vi "ReCalc_V0.15.vi"(3 "Berechnen":bool, 4 "Datenspeicher":T2) -> ()   [LabVIEW 2014]
uses:
  <vilib>/Utility/miscctls.llb/LVPointTypeDef.ctl
  <vilib>/Utility/xml.llb/Read From XML File(string).vi
  <vilib>/Analysis/3filter.llb/IIR Filter (DBL).vi
  <vilib>/Analysis/NI_AALBase.lvlib
  <vilib>/Analysis/NI_AALPro.lvlib
panel:
  out "Fahrzeugdaten":string
  out "Überlagerung":bool
  in  "Überlagern":bool
  out "Übersetzung ermitteln aus":T1(ring)
  in  "Speichern":bool
  out "Reifenumfang [m]":dbl=1.222
  out "Getriebe [1:]":dbl=5.343
  out "Zündung [Imp/U]":u8=1
  out "Rollengeber [Inkr/U]":u16=200
  out "Luftdruck [mbar]":dbl=1013.0
  out "Luftfeuchtigkeit [%]":dbl=50.0
  out "Lufttemperatur [°C]":dbl=20.0
  in  "Stopp":bool
  in  "Rollenträgheit [kgm²]":dbl=0.402
  in  "Polynom":u8=15
  in  "Gl. Mittelwert":u8=35
  in  "Differenzenquotient":u8=12
  in  "n vom Gas [1/min]":dbl=5000.0
  out "Rollenumfang [m]":dbl=0.613 format="%.3f"
  out "Datum, Zeit":string
  out "Untersetzung aus:":dbl=2.68 format="%.2f"
  in  "Drucken":bool
  out "Pmax":string
  out "Ergebnis":string
  out "XY-Graph":cluster{dbl[], dbl[]}[](graph)
  in  "Öffnen":bool
  out "korr":dbl
  out "[s]":dbl=5.0
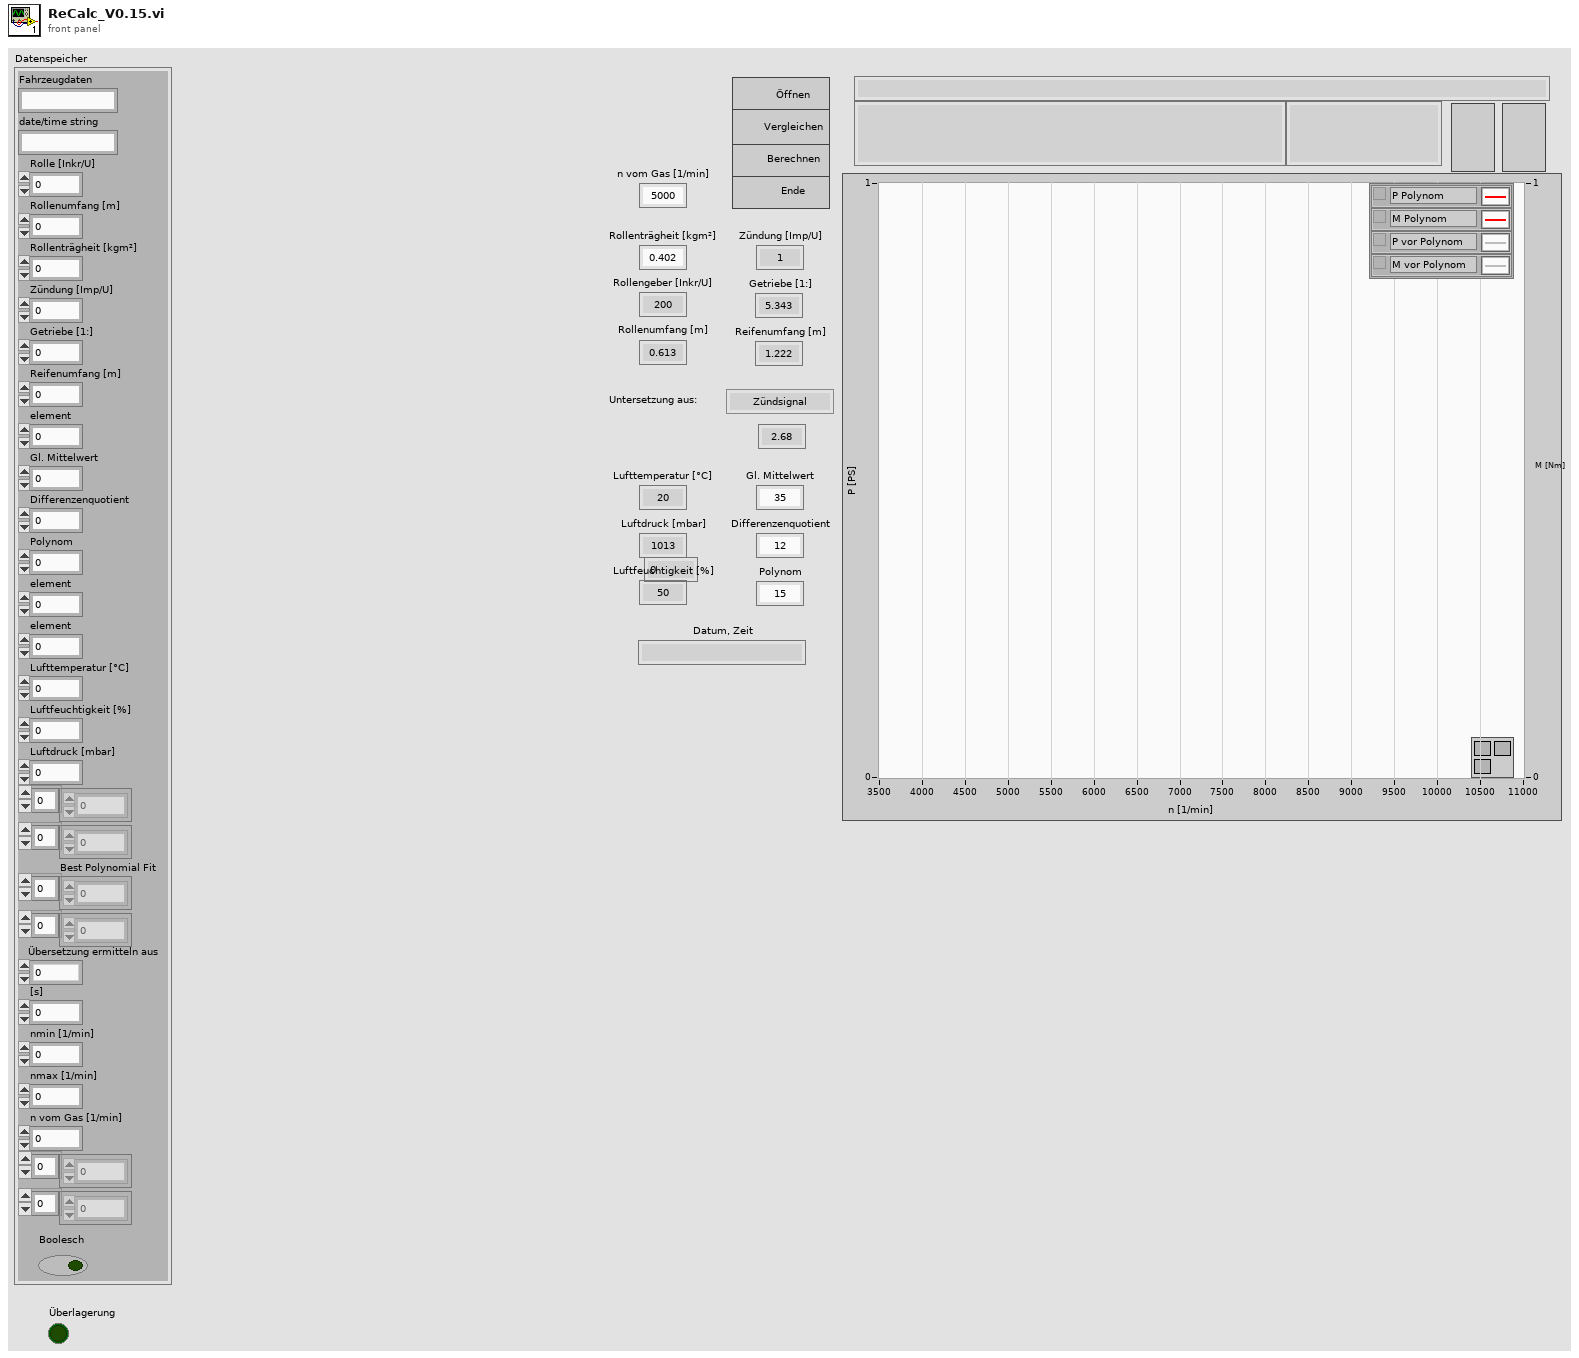
[diagram p1: front panel]
types:
  T1 = enum8{"Zündsignal", "Getriebe & Reifen", "nKuWe / nRolle :"}
  T2 = cluster{"Fahrzeugdaten":string, "date/time string":string, "Rolle [Inkr/U]":u16, "Rollenumfang [m]":dbl, "Rollenträgheit [kgm²]":dbl, "Zündung [Imp/U]":u8, "Getriebe [1:]":dbl, "Reifenumfang [m] ":dbl, "element":dbl, "Gl. Mittelwert":u8, "Differenzenquotient":u8, "Polynom":u8, "element":dbl, "element":dbl, "Lufttemperatur [°C]":dbl, "Luftfeuchtigkeit [%]":dbl, "Luftdruck [mbar]":dbl, dbl[], dbl[], "Best Polynomial Fit":dbl[], dbl[], "Übersetzung ermitteln aus":u8, "[s]":dbl, "nmin [1/min]":dbl, "nmax [1/min]":dbl, "n vom Gas [1/min]":dbl, dbl[], i32[], "Boolesch":bool}
  T3 = typedef "LVPointTypeDef.ctl" = cluster{"Horizontal":i16, "Vertical":i16}
  T4 = enum16{"Kleinste Quadrate", "Kleinestes absolutes Reiduum", "Biquadrat"}
  T5 = enum8{"Enabled", "Disabled", "Disabled and Grayed Out"}
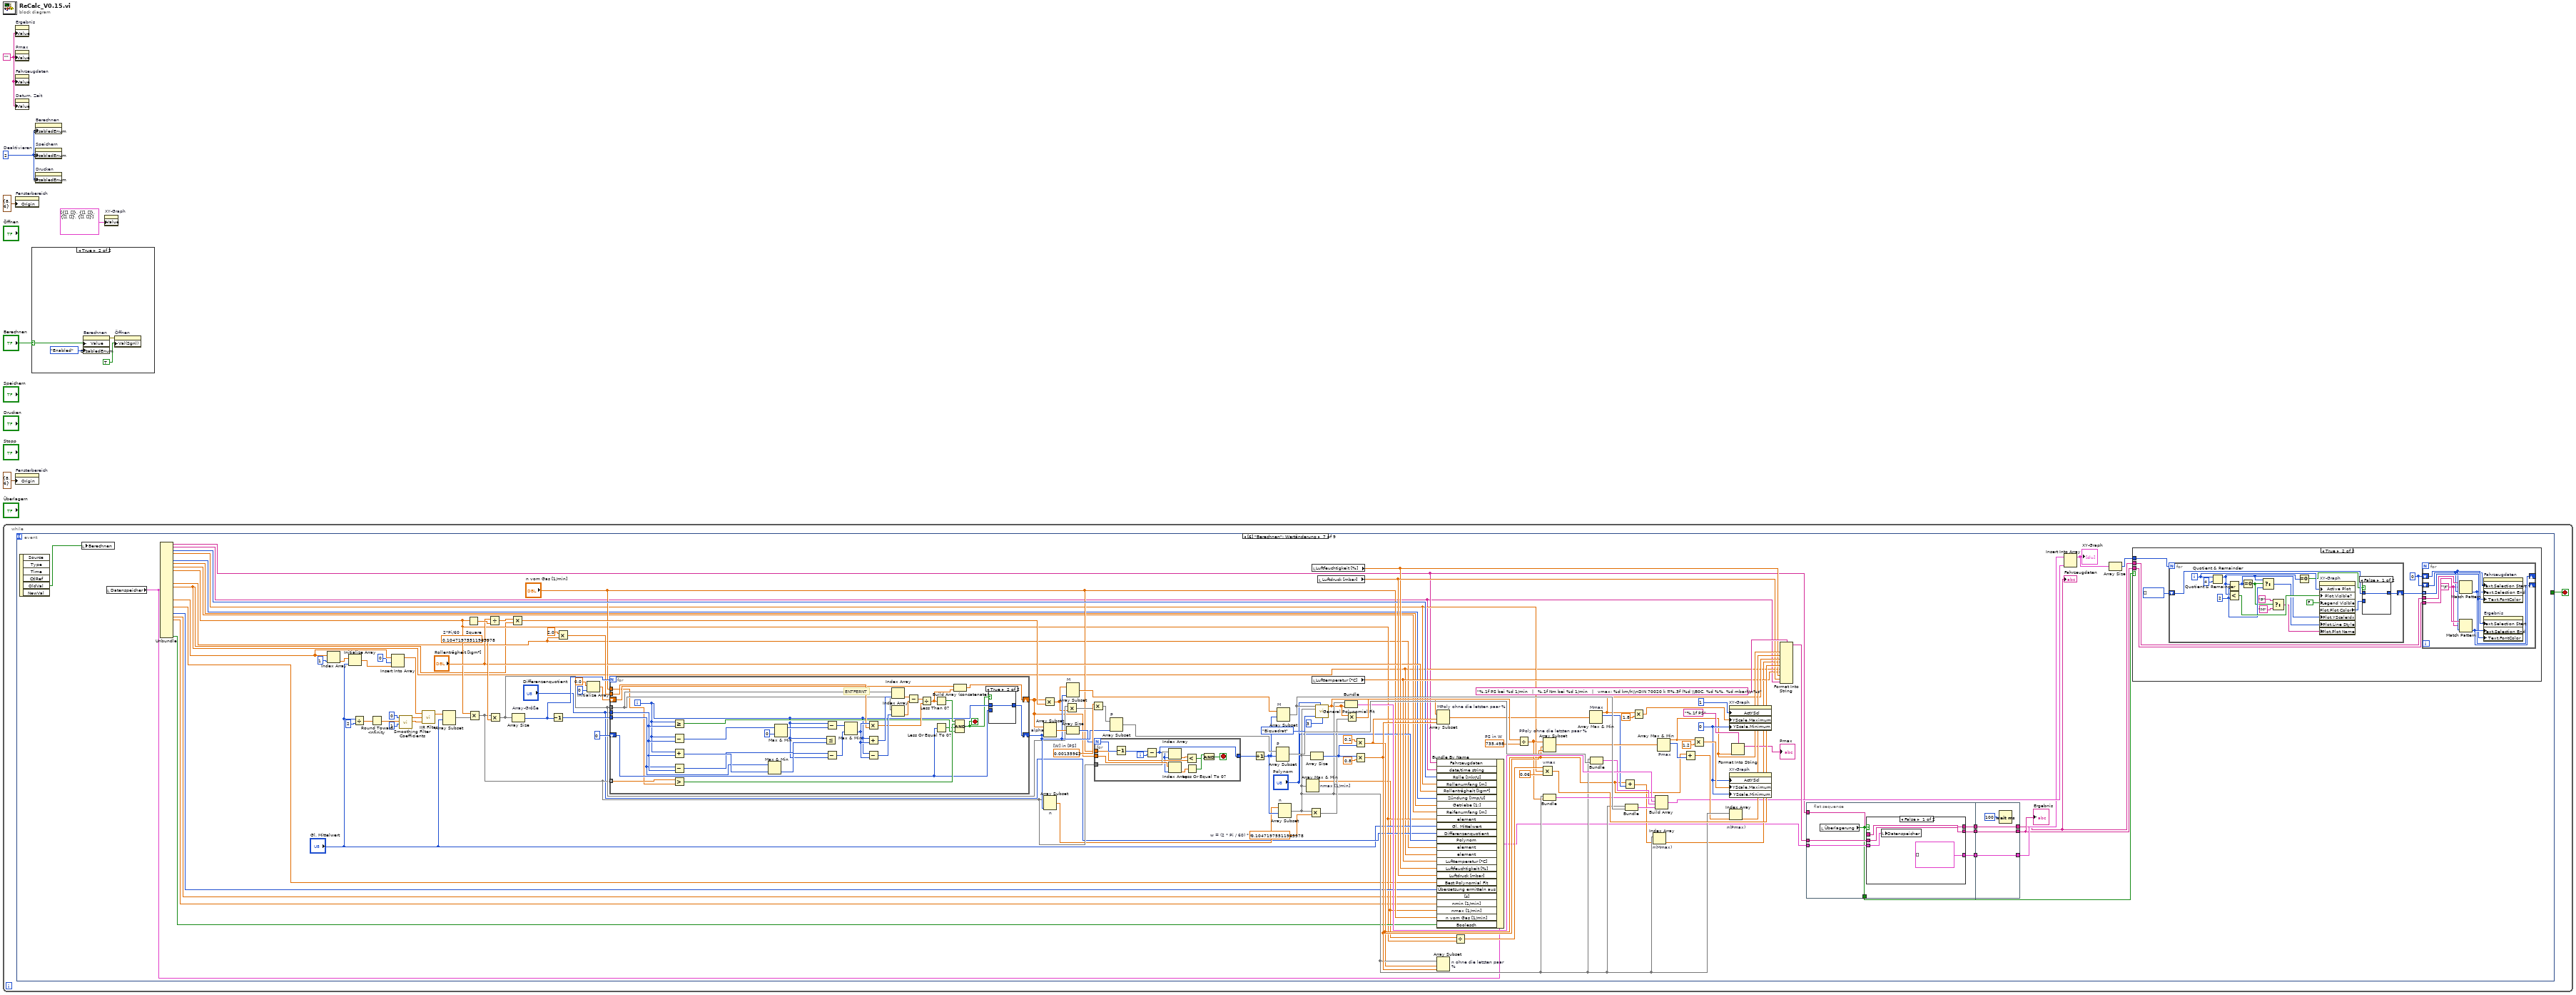
[diagram p0: block diagram]
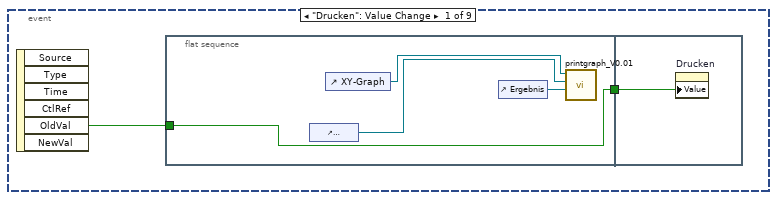
[diagram p3: hidden frame]
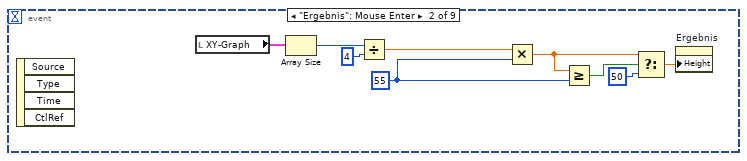
[diagram p4: hidden frame]
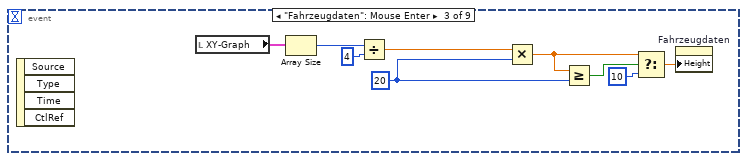
[diagram p5: hidden frame]
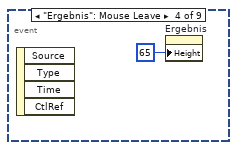
[diagram p6: hidden frame]
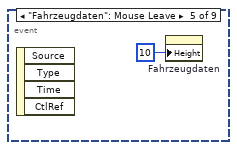
[diagram p7: hidden frame]
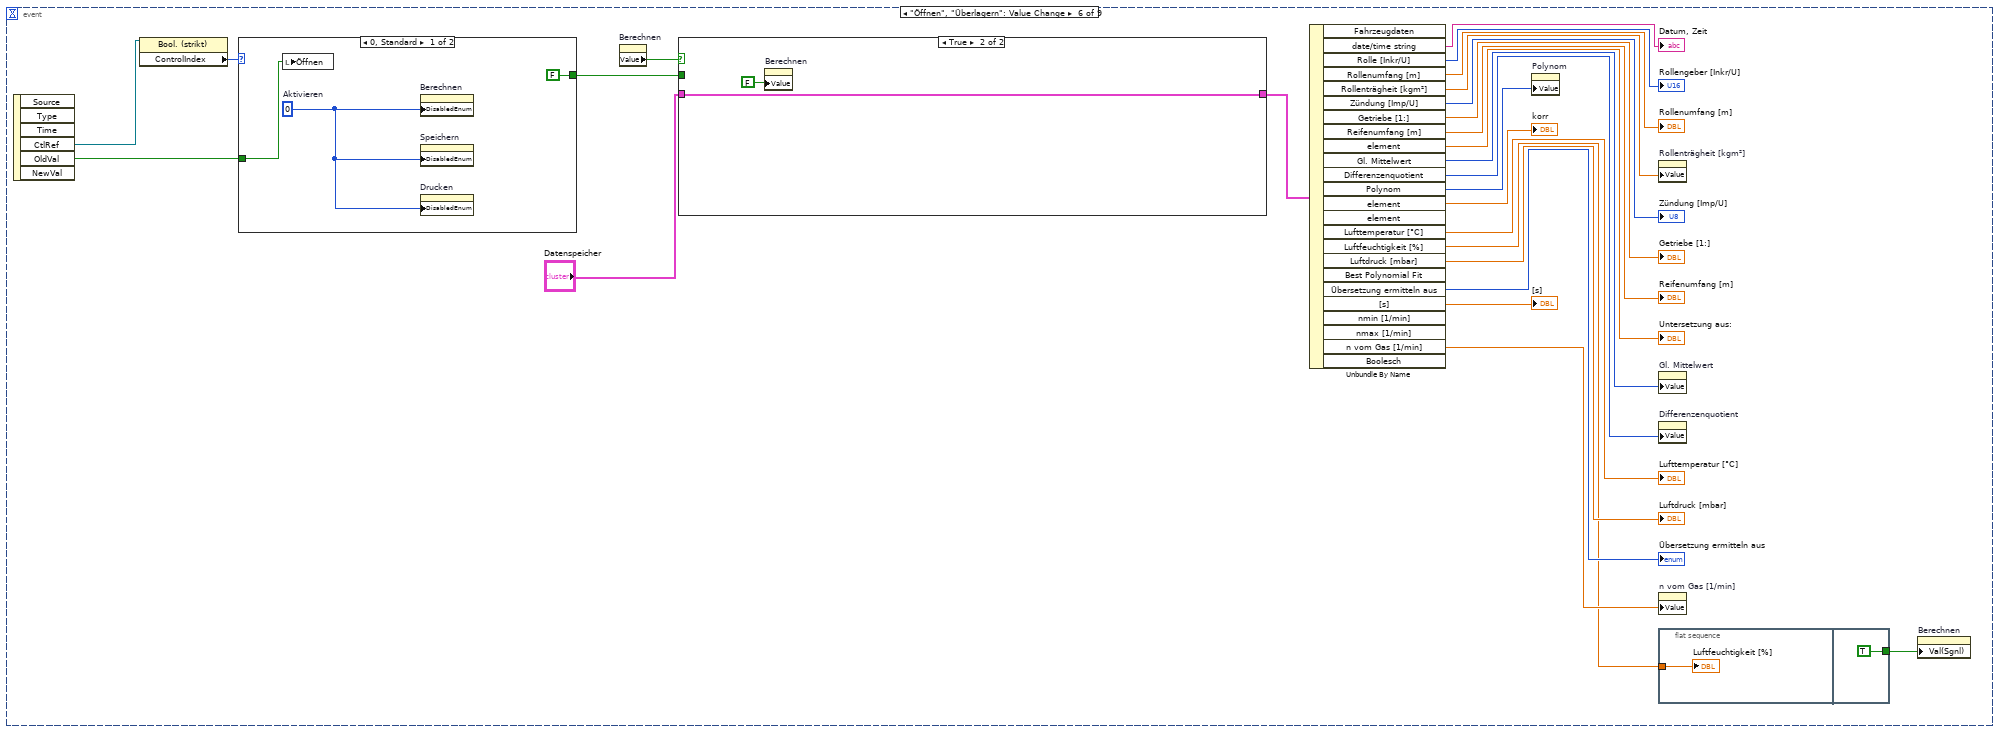
[diagram p8: hidden frame]
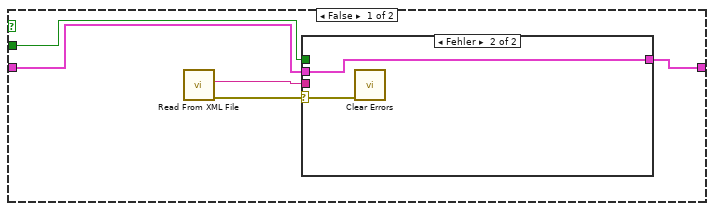
[diagram p9: hidden frame]
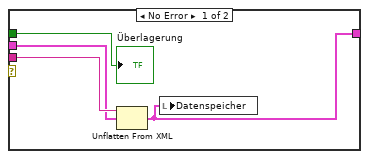
[diagram p10: hidden frame]
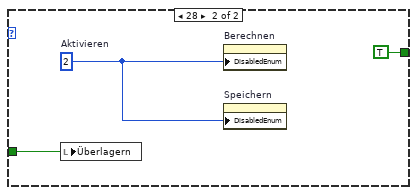
[diagram p11: hidden frame]
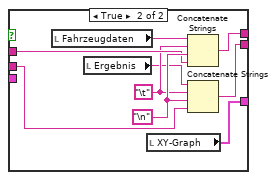
[diagram p12: hidden frame]
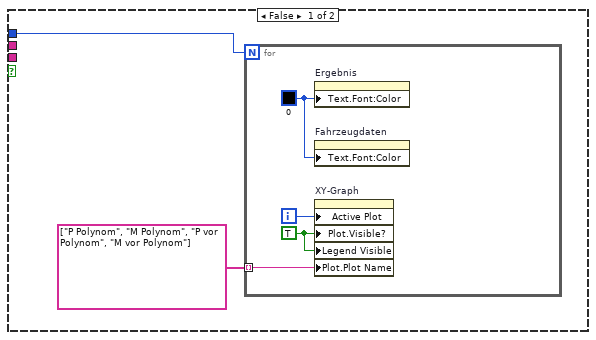
[diagram p13: hidden frame]
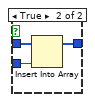
[diagram p14: hidden frame]
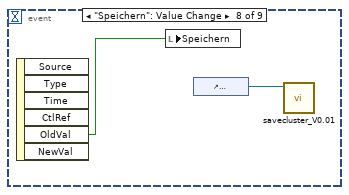
[diagram p16: hidden frame]
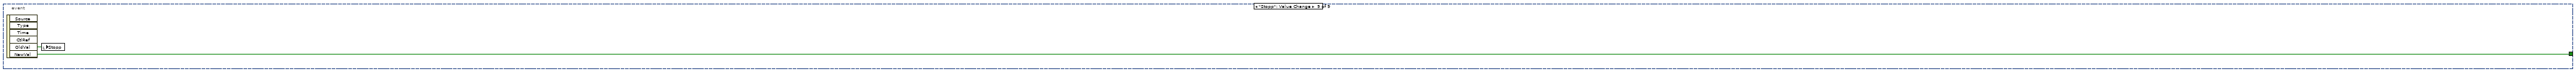
[diagram p17: hidden frame]
diagram:
  w4 = 2  # Deaktivieren
  w6 = ""
  n1 = while {
    stop <- w7 stop-if-true
    n2 = event shown="[6] \"Berechnen\": Wertänderung" {
      selector: _ -> [_ _ _ _ _ _ _ _ _]
      dyn-events: _ -> [_ _ _ _ _ _ _ _ _]
      timeout: _ -> [_ _ _ _ _ _ _ _ _]
      tunnel: [_ _ _ _ _ _ _ _ w317] -> w7
      event "Drucken": Value Change {
        n3 = event-data() -> ("OldVal"=w9:bool)  [unwired: 1 in, 5 out]
        n4 = flat-sequence {
          tunnel: w9 -> [w13]
          tunnel: [w13] -> w8
          tunnel: w8 -> [w14]
          frame #0 {
            n5 = control-ref of="Fahrzeugdaten"() -> (w11:refnum<vi>)
            n6 = control-ref of="XY-Graph"() -> (w12:refnum<vi>)
            n7 = control-ref of="Ergebnis"() -> (w10:refnum<vi>)
            n8 = call "printgraph_V0.01.vi"("reference 2"=w10, "Fahrzeugdaten"=w11, "XYGraph (Eingang)"=w12) -> ()  [unwired: 9 in]
          }
          frame #1 {
            n9 = property on="Drucken" class="Bool. (strikt)"("Value"=w14) -> ()  [unwired: 2 in, 2 out]
          }
        }
      }
      event "Ergebnis": Mouse Enter {
        w17 = u32 55 ("Größe:Höhe")
        n10 = event-data() -> ()  [unwired: 1 in, 4 out]
        n11 = local read "XY-Graph"() -> (w23:cluster{dbl[], dbl[]}[])
        n12 = Array Size(array=w23) -> (size(s)=w22:i32)
        n13 = Divide(x=w22, y=4) -> (x/y=w20:dbl)
        n14 = Multiply(x=w20, y=w17) -> (x*y=w18:dbl)
        n15 = Greater Or Equal?(x=w18, y=w17) -> (x >= y?=w19:bool)
        n16 = Select(t=w18, s=w19, f=u32 50 ("Größe:Höhe")) -> (s? t:f=w16:dbl)
        n17 = property on="Ergebnis" class="Str"("Height"=w16) -> ()  [unwired: 2 in, 2 out]
      }
      event "Fahrzeugdaten": Mouse Enter {
        w26 = u32 20 ("Größe:Höhe")
        n18 = event-data() -> ()  [unwired: 1 in, 4 out]
        n19 = local read "XY-Graph"() -> (w32:cluster{dbl[], dbl[]}[])
        n20 = Array Size(array=w32) -> (size(s)=w31:i32)
        n21 = Divide(x=w31, y=4) -> (x/y=w29:dbl)
        n22 = Multiply(x=w29, y=w26) -> (x*y=w27:dbl)
        n23 = Greater Or Equal?(x=w27, y=w26) -> (x >= y?=w28:bool)
        n24 = Select(t=w27, s=w28, f=u32 10 ("Größe:Höhe")) -> (s? t:f=w25:dbl)
        n25 = property on="Fahrzeugdaten" class="Str"("Height"=w25) -> ()  [unwired: 2 in, 2 out]
      }
      event "Ergebnis": Mouse Leave {
        n26 = event-data() -> ()  [unwired: 1 in, 4 out]
        n27 = property on="Ergebnis" class="Str"("Height"=u32 65 ("Größe:Höhe")) -> ()  [unwired: 2 in, 2 out]
      }
      event "Fahrzeugdaten": Mouse Leave {
        n28 = event-data() -> ()  [unwired: 1 in, 4 out]
        n29 = property on="Fahrzeugdaten" class="Str"("Height"=u32 10 ("Größe:Höhe")) -> ()  [unwired: 2 in, 2 out]
      }
      event "Öffnen", "Überlagern": Value Change {
        n30 = event-data() -> ("CtlRef"=w59:refnum<vi>, "OldVal"=w57:bool)  [unwired: 1 in, 4 out]
        n31 = property class="Bool. (strikt)"(reference=w59) -> ("ControlIndex"=w58:i32)  [unwired: 1 in, 2 out]
        n32 = case shown="0, Standard" w58 {
          tunnel: w57 -> [w78 w81]
          tunnel: [FALSE ("Überlagerung") TRUE ("Überlagerung")] -> w56
          frame 0, Default {
            w76 = 0  # Aktivieren
            n33 = local write "Öffnen"(w78) -> ()
            n34 = property on="Berechnen" class="Bool. (strikt)"("DisabledEnum"=w76) -> ()  [unwired: 2 in, 2 out]
            n35 = property on="Speichern" class="Bool. (strikt)"("DisabledEnum"=w76) -> ()  [unwired: 2 in, 2 out]
            n36 = property on="Drucken" class="Bool. (strikt)"("DisabledEnum"=w76) -> ()  [unwired: 2 in, 2 out]
          }
          frame 28 {
            w79 = 2  # Aktivieren
            n37 = local write "Überlagern"(w81) -> ()
            n38 = property on="Berechnen" class="Bool. (strikt)"("DisabledEnum"=w79) -> ()  [unwired: 2 in, 2 out]
            n39 = property on="Speichern" class="Bool. (strikt)"("DisabledEnum"=w79) -> ()  [unwired: 2 in, 2 out]
          }
        }
        n40 = property on="Berechnen" class="Bool. (strikt)"() -> ("Value"=w35:bool)  [unwired: 2 in, 2 out]
        n41 = case shown="True" w35 {
          tunnel: "Datenspeicher" -> [w64 w72]
          tunnel: w56 -> [w62 _]
          tunnel: [w61 w72] -> w36
          frame False {
            n42 = call-poly <vilib>:"Read From XML File.vi"() -> ("error out"=w63:errorcluster, "XML Elements"=w65:string)  [unwired: 9 in, 1 out]
            n43 = case shown="Fehler" w63 {
              selector: w63 -> [_ w71]
              tunnel: w65 -> [w69 _]
              tunnel: w64 -> [w67 w70]
              tunnel: w62 -> [w68 _]
              tunnel: [w66 w70] -> w61
              frame No Error {
                n44 = Unflatten From XML(xml string=w69, type=w67) -> (value=w66:T2)  [unwired: 1 in, 1 out]
                n45 = local write "Datenspeicher"(w66) -> ()
                "Überlagerung" <- w68
              }
              frame Error {
                n46 = call <vilib>:"Clear Errors.vi"("error in (no error)"=w71) -> ()  [unwired: 5 in, 2 out]
              }
            }
          }
          frame True {
            n47 = property on="Berechnen" class="Bool. (strikt)"("Value"=FALSE) -> ()  [unwired: 2 in, 2 out]
          }
        }
        n48 = Unbundle By Name(w36) -> ("date/time string"=→"Datum, Zeit":string, "Rolle [Inkr/U]"=→"Rollengeber [Inkr/U]":u16, "Rollenumfang [m]"=→"Rollenumfang [m]":dbl, "Rollenträgheit [kgm²]"=w41:dbl, "Zündung [Imp/U]"=→"Zündung [Imp/U]":u8, "Getriebe [1:]"=→"Getriebe [1:]":dbl, "Reifenumfang [m]"=→"Reifenumfang [m]":dbl, "element"=→"Untersetzung aus:":dbl, "Gl. Mittelwert"=w46:u8, "Differenzenquotient"=w47:u8, "Polynom"=w48:u8, "element"=→"korr":dbl, "Lufttemperatur [°C]"=→"Lufttemperatur [°C]":dbl, "Luftfeuchtigkeit [%]"=w51:dbl, "Luftdruck [mbar]"=→"Luftdruck [mbar]":dbl, "Übersetzung ermitteln aus"=→"Übersetzung ermitteln aus":u8, "[s]"=→"[s]":dbl, "n vom Gas [1/min]"=w55:dbl)  [unwired: 6 out]
        n49 = property on="Polynom" class="DigWert (strikt)"("Value"=w48) -> ()  [unwired: 2 in, 2 out]
        n50 = property on="Rollenträgheit [kgm²]" class="DigWert (strikt)"("Value"=w41) -> ()  [unwired: 2 in, 2 out]
        n51 = property on="Gl. Mittelwert" class="DigWert (strikt)"("Value"=w46) -> ()  [unwired: 2 in, 2 out]
        n52 = property on="Differenzenquotient" class="DigWert (strikt)"("Value"=w47) -> ()  [unwired: 2 in, 2 out]
        n53 = property on="n vom Gas [1/min]" class="DigWert (strikt)"("Value"=w55) -> ()  [unwired: 2 in, 2 out]
        n54 = flat-sequence {
          tunnel: w51 -> [w74]
          tunnel: [TRUE] -> w37
          frame #0 {
            "Luftfeuchtigkeit [%]" <- w74
          }
          frame #1 {
          }
        }
        n55 = property on="Berechnen" class="Bool. (strikt)"("Val(Sgnl)"=w37) -> ()  [unwired: 2 in, 2 out]
      }
      event "Berechnen": Value Change {
        w164 = 0
        w172 = 735.498  # PS in W
        w177 = 0.10471975511965978  # w = (2 * Pi / 60) * n
        w188 = 0.00135962  # [W] in [PS]
        w197 = 0.10471975511965978  # 2*Pi/60
        n56 = event-data() -> ("OldVal"=w94:bool)  [unwired: 1 in, 5 out]
        n57 = local write "Berechnen"(w94) -> ()
        n58 = local read "Datenspeicher"() -> (w120:T2)
        n59 = Unbundle(w120) -> ("Fahrzeugdaten"=w86:string, "date/time string"=w85:string, "Rolle [Inkr/U]"=w116:u16, "Rollenumfang [m]"=w107:dbl, "Zündung [Imp/U]"=w106:u8, "Getriebe [1:]"=w105:dbl, "Reifenumfang [m]"=w104:dbl, "element"=w103:dbl, "element"=w102:dbl, "element"=w101:dbl, w203:dbl[], "Best Polynomial Fit"=w100:dbl[], "Übersetzung ermitteln aus"=w108:u8, "[s]"=w97:dbl, "nmin [1/min]"=w98:dbl, "Boolesch"=w111:bool)  [unwired: 13 out]
        n60 = Index Array(array=w203, index=1) -> (element=w126:dbl)
        n61 = Initialize Array(w126, "Gl. Mittelwert") -> (w127:dbl[])
        n62 = Divide(x="Gl. Mittelwert", y=2) -> (x/y=w200:dbl)
        n63 = Round Toward -Infinity(1:w200) -> (0:w199:dbl)
        n64 = Insert Into Array ("In Array einfügen")(array=w203, index=0, new element=w127) -> (w124:dbl[])
        n65 = call <vilib>:"Smoothing Filter Coefficients.vi"("shape"=1, "half-width"=w199, "type"=0) -> ("forward coefficients"=w128:dbl[], "reverse coefficients"=w129:dbl[])  [unwired: 6 in, 1 out]
        n66 = call-poly <vilib>:"IIR Filter.vi"("Forward Coefficients"=w128, "Reverse Coefficients"=w129, "X"=w124) -> ("Filtered X"=w123:dbl[])  [unwired: 1 in, 1 out]
        n67 = Array Subset(array=w123, index="Gl. Mittelwert") -> (w122:dbl[])  [unwired: 1 in]
        n68 = Square(x=w103) -> (x^2=w189:dbl)
        n69 = Multiply(x=w103, y=w122) -> (x*y=w131:dbl[])
        n70 = Divide(x="Rollenträgheit [kgm²]", y=w189) -> (x/y=w186:dbl)
        n71 = Multiply(x=w131, y=w197) -> (x*y=w154:dbl[])
        n72 = Multiply(x=w186, y=w101) -> (x*y=w185:dbl)
        n73 = Array Size "Array-Größe"(array=w154) -> (size(s)=w195:i32)
        n74 = Decrement(x=w195) -> (x-1=w196:i32)
        n75 = Multiply(x=2.0, y=w102) -> (x*y=w194:dbl)
        n76 = Initialize Array(0.0 ("y"), 0) -> (w190:dbl[])
        n77 = for {
          N: w195 -> [_]
          tunnel: "Differenzenquotient" -> [w290]
          tunnel: w154 -> [w297]
          tunnel: w196 -> [w289]
          tunnel: w194 -> [w298]
          shift-right: [w294] -> w153
          shift-left: w190 -> [w295]
          tunnel: w131 -> [w292] mode=indexing
          tunnel: "n vom Gas [1/min]" -> [w281]
          shift-right: [w280] -> w181
          shift-left: 0 -> [w283]
          i -> [w284]
          stop <- w282 stop-if-true
          # "ENTFERNT"
          n78 = Greater Or Equal?(x=w284, y=w290) -> (x >= y?=w287:bool)
          n79 = Subtract(x=w284, y=w290) -> (x-y=w311:i32)
          n80 = Add(x=w284, y=w290) -> (x+y=w305:i32)
          n81 = Subtract(x=w289, y=w290) -> (x-y=w291:i32)
          n82 = Greater?(x=w292, y=w281) -> (0:w293:bool)
          n83 = Max & Min(x=w289, y=w305) -> (min(x,y)=w306:i32)  [unwired: 1 out]
          n84 = Max & Min(x=w311, y=0) -> (max(x,y)=w309:i32)  [unwired: 1 out]
          n85 = Less Or Equal?(x=w284, y=w291) -> ()  [unwired: 1 out]
          n86 = Subtract(x=w284, y=w309) -> (x-y=w308:i32)
          n87 = Subtract(x=w306, y=w284) -> (x-y=w307:i32)
          n88 = Max & Min(x=w308, y=w307) -> (min(x,y)=w299:i32)  [unwired: 1 out]
          n89 = Multiply(x=w299, y=w298) -> (x*y=w296:dbl)
          n90 = Add(x=w284, y=w299) -> (x+y=w304:i32)
          n91 = Subtract(x=w284, y=w299) -> (x-y=w303:i32)
          n92 = Index Array(array=w297, index=w304) -> (element=w301:dbl)
          n93 = Index Array(array=w297, index=w303) -> (element=w302:dbl)
          n94 = Subtract(x=w301, y=w302) -> (x-y=w300:dbl)
          n95 = Divide(x=w300, y=w296) -> (x/y=w288:dbl)
          n96 = Less Than 0?(x=w288) -> (x < 0?=w286:bool)
          n97 = Less Or Equal To 0?(x=w283) -> (x <= 0?=w285:bool)
          n98 = Build Array (concatenate)(w295, w288) -> (w294:dbl[])
          n99 = Compound Arithmetic op=AND(w286, w293, w285, w287) -> (w282:bool)
          n100 = case shown="True" w282 {
            tunnel: w284 -> [_ w313]
            tunnel: [w312 w313] -> w280
            tunnel: w283 -> [w312 _]
            frame False {
            }
            frame True {
            }
          }
        }
        n101 = Multiply(x=w153, y=w185) -> (x*y=w151:dbl[])
        n102 = Array Subset "alpha"(array=w153, length=w181) -> (w183:dbl[])  [unwired: 1 in]
        n103 = Array Subset "n"(array=w131, length=w181) -> (w130:dbl[])  [unwired: 1 in]
        n104 = Multiply(x=w154, y=w151) -> (x*y=w187:dbl[])
        n105 = Array Subset "M"(array=w151, length=w181) -> (w152:dbl[])  [unwired: 1 in]
        n106 = Array Size(array=w183) -> (size(s)=w180:i32)
        n107 = Multiply(x=w188, y=w187) -> (x*y=w182:dbl[])
        n108 = for {
          N: w180 -> [w279]
          tunnel: w153 -> [w276]
          tunnel: w131 -> [w273]
          tunnel: "n vom Gas [1/min]" -> [w270]
          tunnel: [w268] -> w179
          i -> [w274]
          stop <- w269 stop-if-true
          n109 = Decrement(x=w279) -> (x-1=w278:i32)
          n110 = Subtract(x=w278, y=w274) -> (x-y=w268:i32)
          n111 = Index Array(array=w273, index=w268) -> (element=w272:dbl)
          n112 = Index Array(array=w276, index=w268) -> (element=w277:dbl)
          n113 = Less?(x=w272, y=w270) -> (x < y?=w271:bool)
          n114 = Less Or Equal To 0?(x=w277) -> (x <= 0?=w275:bool)
          n115 = And(x=w275, y=w271) -> (x .and. y?=w269:bool)
        }
        n116 = Array Subset "P"(array=w182, length=w181) -> (w171:dbl[])  [unwired: 1 in]
        n117 = Increment(x=w179) -> (x+1=w170:i32)
        n118 = Array Subset "P"(array=w171, index=w170) -> (w178:dbl[])  [unwired: 1 in]
        n119 = Array Subset "M"(array=w152, index=w170) -> (w176:dbl[])  [unwired: 1 in]
        n120 = Array Subset "n"(array=w130, index=w170) -> (w139:dbl[])  [unwired: 1 in]
        n121 = Array Max & Min "nmax [1/min]"(array=w139) -> (max value=w99:dbl)  [unwired: 3 out]
        n122 = Multiply(x=w139, y=w177) -> (x*y=w163:dbl[])
        n123 = Array Size(array=w139) -> (size(s)=w141:i32)
        n124 = local read "Luftfeuchtigkeit [%]"() -> (w118:dbl)
        n125 = local read "Lufttemperatur [°C]"() -> (w117:dbl)
        n126 = call <vilib>:"General Polynomial Fit.vi"("Y"=w176, "polynomial order"="Polynom", "X"=w139, "method"=T4."Biquadrat" ("Methode"), "algorithm"=3) -> ("Best Polynomial Fit"=w138:dbl[])  [unwired: 7 in, 3 out]
        n127 = local read "Luftdruck [mbar]"() -> (w119:dbl)
        n128 = Bundle(w139, "Best Polynomial Fit"=w138) -> (w149:cluster{dbl[], "Best Polynomial Fit":dbl[]})  [unwired: 1 in]
        n129 = Multiply(x=w138, y=w163) -> (x*y=w173:dbl[])
        n130 = Multiply(x=0.1, y=w141) -> (x*y=w134:dbl)
        n131 = Multiply(x=w141, y=0.8) -> (x*y=w142:dbl)
        n132 = Array Subset "MPoly ohne die letzten paar %"(array=w138, index=w134, length=w142) -> (w143:dbl[])
        n133 = Bundle By Name(cluster=w120, "Fahrzeugdaten"=w86, "date/time string"=w85, "Rolle [Inkr/U]"=w116, "Rollenumfang [m]"=w107, "Rollenträgheit [kgm²]"="Rollenträgheit [kgm²]", "Zündung [Imp/U]"=w106, "Getriebe [1:]"=w105, "Reifenumfang [m]"=w104, "element"=w103, "Gl. Mittelwert"="Gl. Mittelwert", "Differenzenquotient"="Differenzenquotient", "Polynom"="Polynom", "element"=w102, "element"=w101, "Lufttemperatur [°C]"=w117, "Luftfeuchtigkeit [%]"=w118, "Luftdruck [mbar]"=w119, "Best Polynomial Fit"=w100, "Übersetzung ermitteln aus"=w108, "[s]"=w97, "nmin [1/min]"=w98, "nmax [1/min]"=w99, "n vom Gas [1/min]"="n vom Gas [1/min]", "Boolesch"=w111) -> (w92:T2)
        n134 = Array Subset "n ohne die letzten paar %"(array=w139, index=w134, length=w142) -> ()  [unwired: 1 out]
        n135 = Divide(x=w99, y=w103) -> (x/y=w162:dbl)
        n136 = Divide(x=w173, y=w172) -> (x/y=w137:dbl[])
        n137 = Array Subset "PPoly ohne die letzten paar %"(array=w137, index=w134, length=w142) -> (w144:dbl[])
        n138 = Compound Arithmetic op=MULTIPLY "vmax"(w162, w107, 0.06) -> (w159:dbl)
        n139 = Bundle(w139, w137) -> (w150:cluster{dbl[], dbl[]})  [unwired: 1 in]
        n140 = Array Max & Min "Mmax"(array=w143) -> (max value=w156:dbl, max index (indices)=w135:i32)  [unwired: 2 out]
        n141 = Bundle(w139, w178) -> (w148:cluster{dbl[], dbl[]})  [unwired: 1 in]
        n142 = Add(x=w134, y=w135) -> (x+y=w133:dbl)
        n143 = Bundle(w139, w176) -> (w147:cluster{dbl[], dbl[]})  [unwired: 1 in]
        n144 = Multiply(x=w156, y=1.8) -> (x*y=w165:dbl)
        n145 = Index Array "n(Mmax)"(array=w139, index=w133) -> (element=w109:dbl)
        n146 = Build Array(w150, w149, w148, w147) -> (w90:cluster{dbl[], "Best Polynomial Fit":dbl[]}[])
        n147 = Array Max & Min "Pmax"(array=w144) -> (max value=w157:dbl, max index (indices)=w136:i32)  [unwired: 2 out]
        n148 = Add(x=w134, y=w136) -> (x+y=w132:dbl)
        n149 = Multiply(x=w157, y=1.2) -> (x*y=w166:dbl)
        n150 = property on="XY-Graph" class="XYGraph (strikt)"("ActYScl"=1, "YScale.Maximum"=w165, "YScale.Minimum"=w164) -> ()  [unwired: 2 in, 2 out]
        n151 = property on="XY-Graph" class="XYGraph (strikt)"("ActYScl"=w164, "YScale.Maximum"=w166, "YScale.Minimum"=w164) -> ()  [unwired: 2 in, 2 out]
        n152 = Index Array "n(Pmax)"(array=w139, index=w132) -> (element=w160:dbl)
        n153 = Format Into String(format string="%.1f PS" ("Format-String"), w157) -> (resulting string=→"Pmax":string)  [unwired: 2 in, 1 out]
        n154 = Format Into String(format string="%.1f PS bei %d 1/min   |   %.1f Nm bei %d 1/min   |   vmax: %d km/h\\nDIN 70020 k =%.3f (%d \\B0C, %d %%, %d mbar)\\n%s" ("Format-String"), w157, w160, w156, w109, w159, w101, w117, w118, w119, w85) -> (resulting string=w96:string)  [unwired: 2 in, 1 out]
        n155 = flat-sequence {
          tunnel: w96 -> [w210]
          tunnel: w92 -> [w209]
          tunnel: [w208] -> w91
          tunnel: w86 -> [w204]
          tunnel: [w207] -> w84
          tunnel: [w206] -> w83
          tunnel: [w205] -> w82
          tunnel: [w225] -> w87
          tunnel: [w226] -> w88
          tunnel: [w227] -> w89
          tunnel: w84 -> [w227]
          tunnel: w83 -> [w226]
          tunnel: w82 -> [w225]
          frame #0 {
            n156 = local read "Überlagerung"() -> (w208:bool)
            n157 = case shown="False" w208 {
              tunnel: [cluster{dbl[], dbl[]}[] [] ("XY-Graph") w223] -> w207
              tunnel: w210 -> [w213 w221]
              tunnel: [w213 w222] -> w206
              tunnel: w209 -> [w212 _]
              tunnel: w204 -> [w211 w219]
              tunnel: [w211 w218] -> w205
              frame False {
                n158 = local write "Datenspeicher"(w212) -> ()
              }
              frame True {
                w217 = "\t"
                w220 = "\n"
                n159 = local read "Fahrzeugdaten"() -> (w216:string)
                n160 = local read "Ergebnis"() -> (w215:string)
                n161 = local read "XY-Graph"() -> (w223:cluster{dbl[], dbl[]}[])
                n162 = Concatenate Strings(w216, w217, w220, w219) -> (w218:string)
                n163 = Concatenate Strings(w215, w217, w220, w221) -> (w222:string)
              }
            }
          }
          frame #1 {
            n164 = Wait (ms)(milliseconds to wait=u32 100 ("Zu wartende ms")) -> ()  [unwired: 1 out]
          }
        }
        n165 = Insert Into Array(array=w89, new element=w90) -> (w93:cluster{dbl[], dbl[]}[])  [unwired: 1 in]
        "XY-Graph" <- w93
        n166 = Array Size(array=w93) -> (size(s)=w95:i32)
        n167 = case shown="True" w91 {
          tunnel: w95 -> [w229 w239]
          tunnel: w88 -> [_ w236]
          tunnel: w87 -> [_ w235]
          frame False {
            n168 = for {
              N: w229 -> [_]
              tunnel: string[] ["P Polynom", "M Polynom", "P vor Polynom", "M vor Polynom"] -> [w231] mode=indexing
              i -> [w233]
              w230 = u32 0
              w232 = TRUE ("Plot.Sichtbar")
              n169 = property on="Ergebnis" class="Str"("Text.Font:Color"=w230) -> ()  [unwired: 2 in, 2 out]
              n170 = property on="Fahrzeugdaten" class="Str"("Text.Font:Color"=w230) -> ()  [unwired: 2 in, 2 out]
              n171 = property on="XY-Graph" class="XYGraph (strikt)"("Active Plot"=w233, "Plot.Visible?"=w232, "Legend Visible"=w232, "Plot.Plot Name"=w231) -> ()  [unwired: 2 in, 2 out]
            }
          }
          frame True {
            w234 = 0
            n172 = for {
              N: w239 -> [_]
              shift-right: [w258] -> w237
              shift-left: u32[] [] -> [w257]
              i -> [w262]
              w253 = 2 ("y")
              n173 = Quotient & Remainder(x=w262, y=4) -> (x-y*floor(x/y)=w255:i32)  [unwired: 1 out]
              n174 = Less?(x=w255, y=w253) -> (x < y?=w261:bool)
              n175 = Quotient & Remainder(x=w255, y=w253) -> (x-y*floor(x/y)=w254:i32)  [unwired: 1 out]
              n176 = Equal To 0?(x=w254) -> (x = 0?=w251:bool)
              n177 = Select(t=w254, s=w251, f=w253) -> (s? t:f=w252:i32)
              n178 = Select(t="P" ("Plot.Plotname"), s=w251, f="M" ("Plot.Plotname")) -> (s? t:f=w248:string)
              n179 = Equal To 0?(x=w255) -> (x = 0?=w256:bool)
              n180 = property on="XY-Graph" class="XYGraph (strikt)"("Active Plot"=w262, "Plot.Visible?"=w261, "Legend Visible"=FALSE ("Legende:Sichtbar"), "Plot.YScaleIdx"=w254, "Plot.Line Style"=w252, "Plot.Plot Name"=w248) -> ("Plot.Plot Color"=w259:u32)  [unwired: 2 in, 2 out]
              n181 = case shown="False" w256 {
                tunnel: w259 -> [_ w267]
                tunnel: [w264 w266] -> w258
                tunnel: w257 -> [w264 w265]
                frame False {
                }
                frame True {
                  n182 = Insert Into Array(array=w265, new element=w267) -> (w266:u32[])  [unwired: 1 in]
                }
              }
            }
            n183 = for {
              shift-right: [w247] -> _
              shift-left: w234 -> [w244]
              tunnel: w237 -> [w245] mode=indexing
              tunnel: w236 -> [w246]
              tunnel: w235 -> [w243]
              shift-right: [w242] -> _
              shift-left: w234 -> [w241]
              w240 = "\t"
              n184 = Match Pattern(string=w243, regular expression=w240, offset (0)=w241) -> (offset past match=w242:i32)  [unwired: 3 out]
              n185 = Match Pattern(string=w246, regular expression=w240, offset (0)=w244) -> (offset past match=w247:i32)  [unwired: 3 out]
              n186 = property on="Fahrzeugdaten" class="Str"("Text.Selection Start"=w241, "Text.Selection End"=w242, "Text.FontColor"=w245) -> ()  [unwired: 2 in, 2 out]
              n187 = property on="Ergebnis" class="Str"("Text.Selection Start"=w244, "Text.Selection End"=w247, "Text.FontColor"=w245) -> ()  [unwired: 2 in, 2 out]
            }
          }
        }
        "Ergebnis" <- w88
        "Fahrzeugdaten" <- w87
      }
      event "Speichern": Value Change {
        n188 = event-data() -> ("OldVal"=w315:bool)  [unwired: 1 in, 5 out]
        n189 = local write "Speichern"(w315) -> ()
        n190 = control-ref of="Datenspeicher"() -> (w314:refnum<vi>)
        n191 = call "savecluster_V0.01.vi"("Cluster (Eingang)"=w314) -> ()  [unwired: 11 in]
      }
      event "Stopp": Value Change {
        n192 = event-data() -> ("OldVal"=w316:bool, "NewVal"=w317:bool)  [unwired: 1 in, 4 out]
        n193 = local write "Stopp"(w316) -> ()
      }
    }
  }
  n194 = property on="Ergebnis" class="Str"("Value"=w6) -> ()  [unwired: 2 in, 2 out]
  n195 = property on="Pmax" class="Str"("Value"=w6) -> ()  [unwired: 2 in, 2 out]
  n196 = property on="Fahrzeugdaten" class="Str"("Value"=w6) -> ()  [unwired: 2 in, 2 out]
  n197 = property on="Datum, Zeit" class="Str"("Value"=w6) -> ()  [unwired: 2 in, 2 out]
  n198 = property on="Fensterbereich" class="Bereich"("Origin"=T3 {"Horizontal"=8, "Vertical"=6}) -> ()  [unwired: 2 in, 2 out]
  n199 = property on="Fensterbereich" class="Bereich"("Origin"=T3 {"Horizontal"=8, "Vertical"=6}) -> ()  [unwired: 2 in, 2 out]
  n200 = case shown="True" "Berechnen" {
    selector: "Berechnen" -> [_ w321]
    frame False {
    }
    frame True {
      n201 = property on="Berechnen" class="Bool. (strikt)"("Value"=w321, "DisabledEnum"=T5."Enabled" ("Deaktiviert")) -> (error out=w318:errorcluster)  [unwired: 2 in, 1 out]
      n202 = property on="Öffnen" class="Bool. (strikt)"(error in=w318, "Val(Sgnl)"=TRUE ("Wert (signalisierend)")) -> ()  [unwired: 1 in, 2 out]
    }
  }
  n203 = property on="Berechnen" class="Bool. (strikt)"("DisabledEnum"=w4) -> ()  [unwired: 2 in, 2 out]
  n204 = property on="Speichern" class="Bool. (strikt)"("DisabledEnum"=w4) -> ()  [unwired: 2 in, 2 out]
  n205 = property on="Drucken" class="Bool. (strikt)"("DisabledEnum"=w4) -> ()  [unwired: 2 in, 2 out]
  n206 = property on="XY-Graph" class="XYGraph (strikt)"("Value"=cluster{dbl[], dbl[]}[] [{[], []}, {[], []}, {[], []}, {[], []}] ("XY-Graph")) -> ()  [unwired: 2 in, 2 out]
